vi "cp_algorithm.vi"(4 "CP flag":i32, 5 "1P last":i32[](array[numeric]), 6 "empty":i32[](array[numeric]), 7 "table":i32[](array[numeric])) -> (0 "CP_fin":bool, 1 "hit":i32, 2 "empty out":i32[](array[numeric]), 3 "table out":i32[](array[numeric]))   [LabVIEW 8.6]
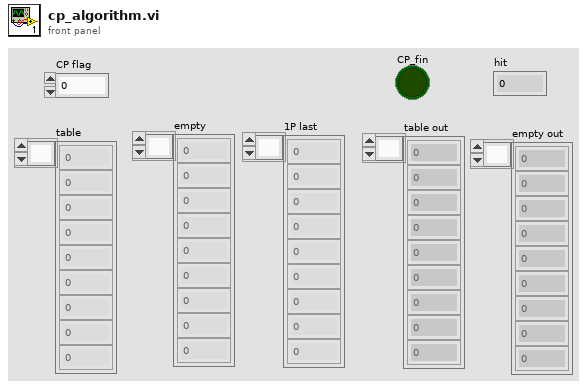
[diagram p1: front panel]
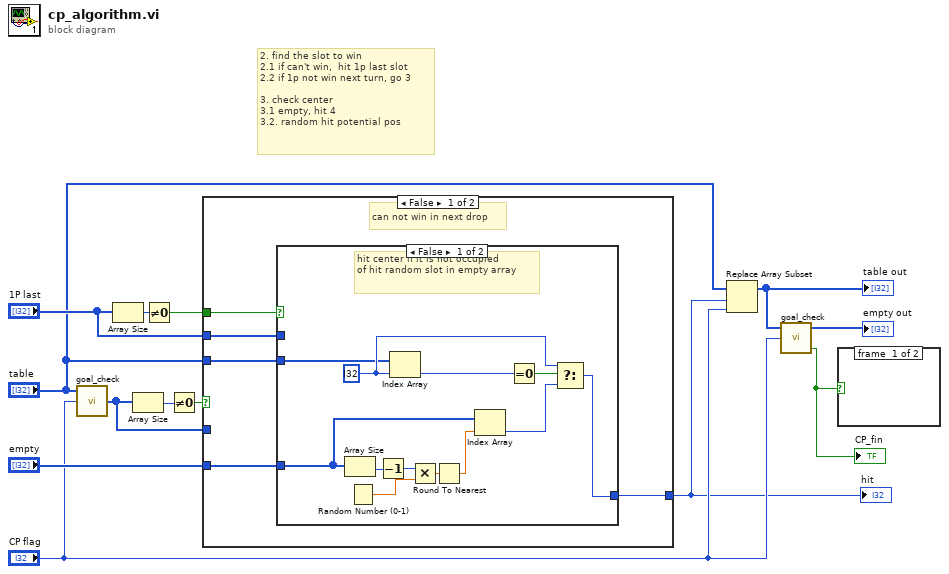
[diagram p0: block diagram]
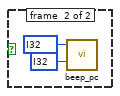
[diagram p2: hidden frame]
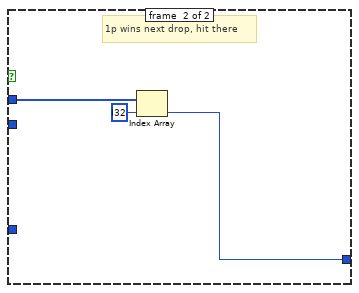
[diagram p3: hidden frame]
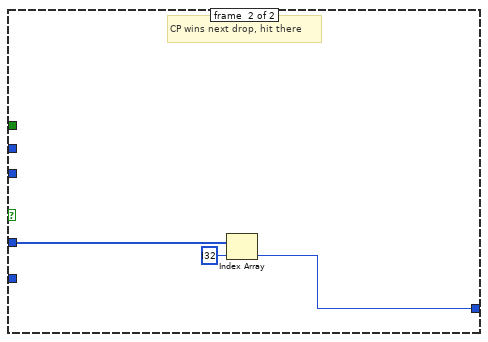
[diagram p4: hidden frame]
diagram:
  # "2. find the slot to win\n2.1 if can't win,  hit 1p last slot\n2.2 if 1p not win next turn, go 3\n\n3. check center\n3.1 empty, hit 4\n3.2. random hit potential pos"
  n1 = call "goal_check.vi"("flag"="CP flag", "table"="table") -> ("win step"=w9:i32[])  [unwired: 1 in, 2 out]
  n2 = Array Size(array="1P last") -> (size(s)=w13:i32)
  n3 = Array Size(array=w9) -> (size(s)=w11:i32)
  n4 = Not Equal To 0?(x=w13) -> (x != 0?=w8:bool)
  n5 = Not Equal To 0?(x=w11) -> (x != 0?=w10:bool)
  n6 = case shown="False" w10 {
    tunnel: "1P last" -> [w18 _]
    tunnel: "table" -> [w17 _]
    tunnel: [w16 w34] -> w3
    tunnel: w9 -> [_ w35]
    tunnel: w8 -> [w15 _]
    tunnel: "empty" -> [w14 _]
    frame #0 {
      # "can not win in next drop"
      n7 = case shown="False" w15 {
        tunnel: w18 -> [_ w31]
        tunnel: w17 -> [w21 _]
        tunnel: [w19 w32] -> w16
        tunnel: w14 -> [w20 _]
        frame #0 {
          w27 = i32 ? ("index")
          # "hit center if it is not occupied\nof hit random slot in empty array"
          n8 = Array Size(array=w20) -> (size(s)=w22:i32)
          n9 = Random Number (0-1)() -> (number: 0 to 1=w24:dbl)
          n10 = Decrement(x=w22) -> (x-1=w23:i32)
          n11 = Index Array(array=w21, index=w27) -> (element=w29:i32)
          n12 = Multiply(x=w23, y=w24) -> (x*y=w25:dbl)
          n13 = Round To Nearest(number=w25) -> (nearest integer value=w26:dbl)
          n14 = Index Array(array=w20, index=w26) -> (element=w30:i32)
          n15 = Equal To 0?(x=w29) -> (x = 0?=w28:bool)
          n16 = Select(t=w27, s=w28, f=w30) -> (s? t:f=w19:i32)
        }
        frame #1 {
          # "1p wins next drop, hit there"
          n17 = Index Array(array=w31, index=i32 ?) -> (element=w32:i32)
        }
      }
    }
    frame #1 {
      # "CP wins next drop, hit there"
      n18 = Index Array(array=w35, index=i32 ?) -> (element=w34:i32)
    }
  }
  "hit" <- w3
  n19 = Replace Array Subset(array="table", new element="CP flag", index=w3) -> (w5:i32[])
  "table out" <- w5
  n20 = call "goal_check.vi"("flag"="CP flag", "table"=w5) -> ("fin"=w1:bool, "empty"=→"empty out":i32[])  [unwired: 1 in, 1 out]
  "CP_fin" <- w1
  n21 = case shown="True" w1 {
    frame #0 {
    }
    frame #1 {
      n22 = call "beep_pc.vi"("Duration (seconds)"=i32 ?, "Frequency (Hz)"=i32 ?) -> ()  [unwired: 2 in, 1 out]
    }
  }
